vi "MenuBuild.vi"(8 "error in (no error)":errorcluster, 9 "Insert Tag":string, 10 "menu reference":refnum<k9>, 11 "InsertFunctionMenu in":refnum<class "InsertFunctionMenu.lvclass">) -> (0 "error out":errorcluster, 2 "menu reference out":refnum<k9>, 3 "InsertFunctionMenu out":refnum<class "InsertFunctionMenu.lvclass">)   [LabVIEW 2013, in "InsertFunctionMenu.lvclass"]
uses:
  InsertFunctionMenu.lvclass
  <vilib>/Utility/error.llb/DialogType.ctl
  InsertFunctionMenu.lvclass/InsertFunctionMenu.ctl
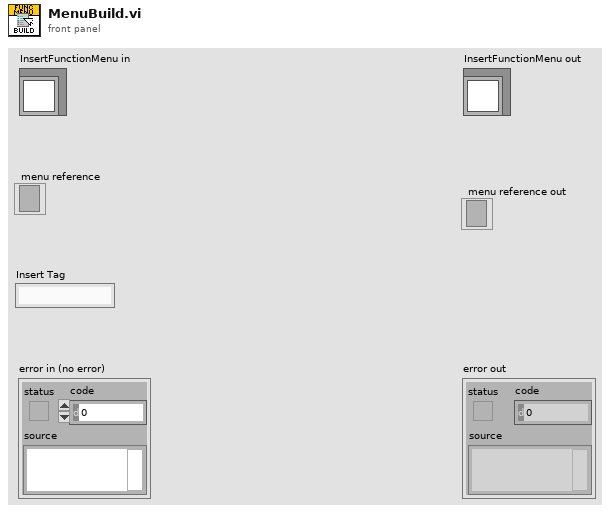
[diagram p1: front panel]
types:
  T1 = typedef "DialogType.ctl" = u16
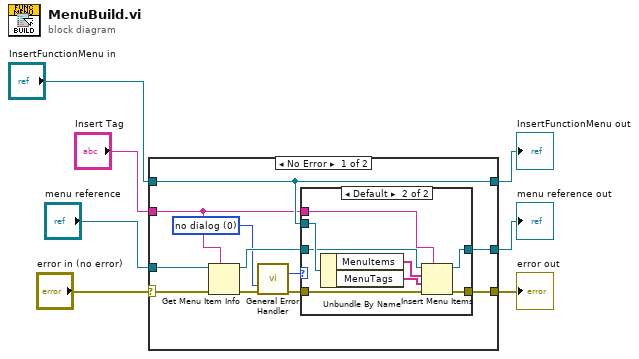
[diagram p0: block diagram]
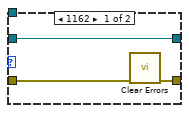
[diagram p2: hidden frame]
diagram:
  n1 = case shown="No Error" "error in (no error)" {
    selector: "error in (no error)" -> [w12 w32]
    tunnel: [w16 w32] -> w6
    tunnel: [w17 w31] -> w4
    tunnel: "InsertFunctionMenu in" -> [w17 w31]
    tunnel: "Insert Tag" -> [w15 _]
    tunnel: "menu reference" -> [w14 w30]
    tunnel: [w18 w30] -> w2
    frame No Error {
      w9 = T1 0 items=["no dialog", "OK message", "continue or stop message", "OK message + warnings", "continue/stop + warnings"] ("type of dialog (OK msg:1)")
      n2 = Get Menu Item Info(7:w15, 8:w12, 11:w14) -> (0:w11:errorcluster, 3:w13:refnum<k9>)  [unwired: 5 out]
      n3 = call <vilib>:"General Error Handler.vi"("type of dialog (OK msg:1)"=w9, "error in (no error)"=w11) -> ("code out"=w8:i32, "error out"=w10:errorcluster)  [unwired: 9 in, 3 out]
      n4 = case shown="Default" w8 {
        tunnel: [w21 w29] -> w18
        tunnel: w17 -> [_ w28]
        tunnel: [w19 w25] -> w16
        tunnel: w15 -> [_ w24]
        tunnel: w13 -> [w21 w23]
        tunnel: w10 -> [w20 w22]
        frame 1162 {
          n5 = call <vilib>:"Clear Errors.vi"("error in (no error)"=w20) -> ("error out"=w19:errorcluster)  [unwired: 6 in]
        }
        frame Default {
          n6 = Unbundle By Name(w28) -> ("MenuItems"=w27:string[], "MenuTags"=w26:string[])
          n7 = Insert Menu Items(5:w24, 6:w22, 7:w26, 8:w27, 9:w23) -> (0:w25:errorcluster, 3:w29:refnum<k9>)  [unwired: 1 in, 1 out]
        }
      }
    }
    frame Error {
    }
  }
  "error out" <- w6
  "InsertFunctionMenu out" <- w4
  "menu reference out" <- w2
